vi "Get Min and Max from Range.vi"(8 "error in (no error)":errorcluster, 11 "BinXRange":refnum<k24>) -> (0 "error out":errorcluster, 1 "Maximum":u32, 2 "Minimum":u32)   [LabVIEW 2022 SP3]
uses:
  I:/.shortcut-targets-by-id/1riZacJd_1_jmKfGgrjDuP7KcecvMS3i2/Xiao research group/Programs/XYZRecorrection/Scientific Camera Interfaces/SDK/DotNet Toolkit/dlls/Managed_64_lib/Thorlabs.TSI.CoreInterfaces.dll
  SDK/DotNet Toolkit/dlls/Managed_64_lib/Thorlabs.TSI.CoreInterfaces.dll
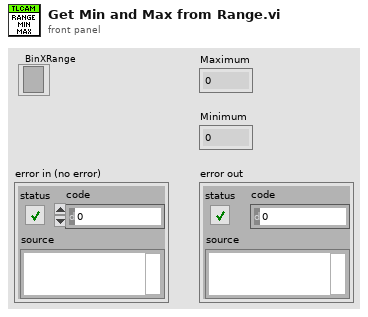
[diagram p1: front panel]
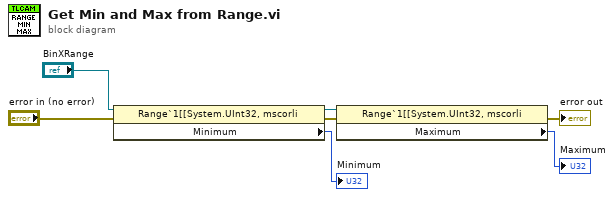
[diagram p0: block diagram]
diagram:
  n1 = property class="Range`1[[System.UInt32, mscorli"(reference="BinXRange", error in="error in (no error)") -> (reference out=w3:refnum<k24>, error out=w4:errorcluster, "Minimum"=→"Minimum":u32)
  n2 = property class="Range`1[[System.UInt32, mscorli"(reference=w3, error in=w4) -> (error out=→"error out":errorcluster, "Maximum"=→"Maximum":u32)  [unwired: 1 out]
